vi "Update Autocomplete.vi"(8 "error in (no error)":errorcluster, 11 "Editor in":refnum<class "Editor.lvclass">) -> (0 "error out":errorcluster, 3 "Editor out":refnum<class "Editor.lvclass">)   [LabVIEW 2020, in "VolatusGUIEditor.lvlib" / "Editor.lvclass"]
uses:
  Editor.lvclass
  Editor.lvclass/Editor.ctl
  lv-volatus/VolatusConfig/VolatusConfig.lvlib
  lv-volatus/VolatusConfig/Meta Type.ctl
  lv-cdm/CDM-Config/Config Filter/Config Lookup.lvclass
  lv-volatus/VolatusConfig/VolatusConfig/VolatusConfig.lvclass
  lv-cdm/CDM-Config/Config Element/Config Element.lvclass
  lv-autocomplete/AutoComplete/Shared Options/Shared Options.lvclass
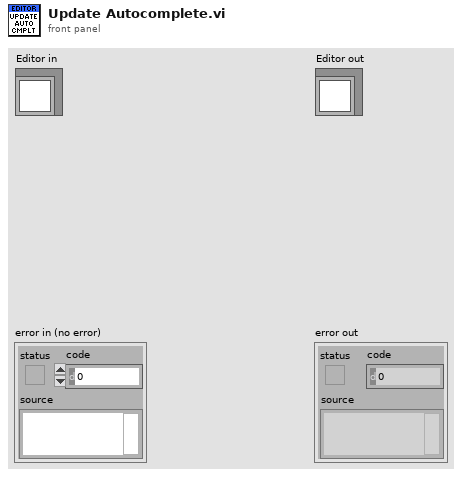
[diagram p1: front panel]
types:
  T1 = typedef "VolatusConfig.lvlib/Meta Type.ctl" = enum16{"UNKNOWN", "VL_System", "VL_Cluster", "VL_Node", "VL_Task", "VL_Group", "VL_Channel", "VL_Task_List", "VL_Scaling", "VL_Sensor", "VL_Sensor_List", "VL_Scale"}
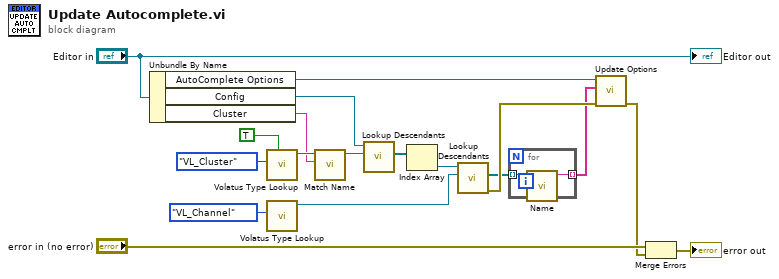
[diagram p0: block diagram]
diagram:
  n1 = Unbundle By Name("Editor in") -> ("AutoComplete Options"=w4:refnum<class "Shared Options.lvclass">, "Config"=w10:refnum<class "VolatusConfig.lvclass">, "Cluster"=w12:string)
  n2 = call "Volatus Type Lookup.vi"("Don't Recurse Past Match (F)"=TRUE, "Meta Type"=Meta_Type."VL_Cluster") -> ("Config Lookup out"=w13:refnum<class "Config Lookup.lvclass">)  [unwired: 8 in, 1 out]
  n3 = call "Volatus Type Lookup.vi"("Meta Type"=Meta_Type."VL_Channel") -> ("Config Lookup out"=w6:refnum<class "Config Lookup.lvclass">)  [unwired: 9 in, 1 out]
  n4 = call "Match Name.vi"("Name"=w12, "Config Lookup (New)"=w13) -> ("Config Lookup out"=w11:refnum<class "Config Lookup.lvclass">)  [unwired: 8 in, 1 out]
  n5 = call "Lookup Descendants.vi"("Lookup"=w11, "VolatusConfig in"=w10) -> ("Descendants"=w9:refnum<class "Config Element.lvclass">[])  [unwired: 7 in, 2 out]
  n6 = Index Array(array=w9) -> (element=w8:refnum<class "Config Element.lvclass">)  [unwired: 1 in]
  n7 = call "Lookup Descendants.vi"("Lookup"=w6, "Config Element in"=w8) -> ("error out"=w18:errorcluster, "Descendants"=w5:refnum<class "Config Element.lvclass">[])  [unwired: 7 in, 1 out]
  n8 = for {
    tunnel: w5 -> [w20] mode=indexing
    tunnel: [w19] -> w3 mode=indexing
    n9 = call "Name.vi"("Config Element in"=w20) -> ("Name"=w19:string)  [unwired: 9 in, 1 out]
  }
  n10 = call "Update Options.vi"("error in (no error)"=w18, "Options"=w3, "Shared Options in"=w4) -> ("error out"=w1:errorcluster)  [unwired: 7 in, 1 out]
  n11 = Merge Errors("error in (no error)", w1) -> (→"error out":errorcluster)
  "Editor out" <- "Editor in"
